vi "打印.vi"(8 "error in (no error)":errorcluster caption="错误输入（无错误）", 11 "Animal 输入":refnum<class "Animal.lvclass">) -> (0 "error out":errorcluster caption="错误输出", 2 "字符串":string, 3 "Animal 输出":refnum<class "Animal.lvclass">)   [LabVIEW 2020, in "Animal.lvclass"]
uses:
  Animal.lvclass
  Animal.lvclass/Animal.ctl
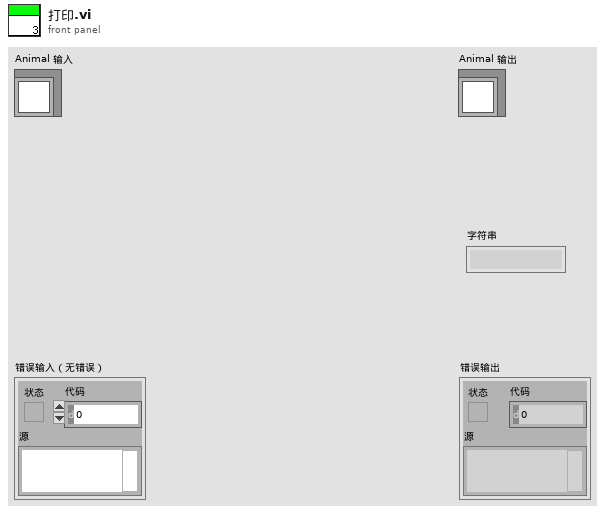
[diagram p1: front panel]
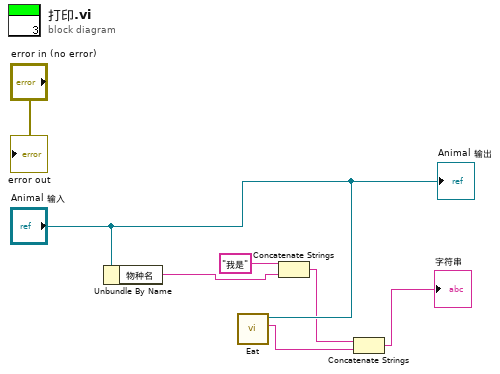
[diagram p0: block diagram]
diagram:
  n1 = Unbundle By Name("Animal 输入") -> ("物种名"=w6:string)
  n2 = call-dynamic "Eat.vi"("Animal 输入"="Animal 输入") -> ("字符串 2"=w3:string)  [unwired: 8 in, 2 out]
  n3 = Concatenate Strings("我是", w6) -> (w4:string)
  n4 = Concatenate Strings(w4, w3) -> (→"字符串":string)
  "error out" <- "error in (no error)"
  "Animal 输出" <- "Animal 输入"
